vi "VI Modbus KOMM .vi"(8 "error in (no error)":errorcluster caption="Fehler (Eingang)") -> (0 "error out":errorcluster caption="Fehler (Ausgang)")   [LabVIEW 2020, in "PNS.lvlib" / "Komm Modbus.lvlib"]
uses:
  Komm Modbus.lvlib
  Aktionen FGV Komm MB.ctl
  Aktionen FGV Istwerte.ctl
  Seiten/System Einstellungen V2/Aktioen FGV System.ctl
  Stoerungen/Stoerungen Messgeraet/Aktionen Kommunikation Stoerung.ctl
  Aktionen FGV Grenzwerte.ctl
  Modbus TypDef.lvlib
  Stoerungen/Stoerungen.lvlib
  PNS.lvlib
  Seiten/System Einstellungen V2/System Einstellungen V2.lvlib
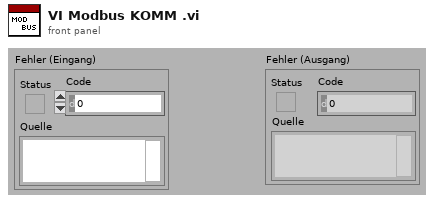
[diagram p1: front panel]
types:
  T1 = typedef "PNS.lvlib/Aktionen FGV Istwerte.ctl" = enum16{"lesen", "initialisieren", "schreiben", "Störungen"}
  T2 = typedef "PNS.lvlib/Komm Modbus.lvlib/Modbus TypDef.lvlib/Aktionen FGV Komm MB.ctl" = enum16{"initialisieren", "lesen", "Verbindung herstellen", "Verbindung beenden", "Komm Modbus", "Sollwerte vorgeben", "change lang"}
  T3 = typedef "System Einstellungen V2.lvlib/Aktioen FGV System.ctl" = enum16{"lesen", "laden", "speichern", "Optionen schreiben", "Zeitstempel", "Reset BMP", "Reset SQP", "Wartung", "Werkseinstellung"}
  T4 = typedef "Stoerungen.lvlib/Aktionen Kommunikation Stoerung.ctl" = enum16{"lesen", "init", "FT-IR Komm", "FT-IR Betriebsart", "FT-IR Hintergrund", "cRIO Komm", "PNS Komm", "Dichtheitstest", "Life Bit", "FTIR Komm AK", "PMA Komm", "FID Komm", "PMA Cal", "FID Ch4 Cal", "FID THC Cal", "Cal Timeout", "VFS 1 Komm", "VFS 2 Komm", "VFS 3 Komm", "VFS 4 Komm", "TRE 08 Komm", "CG-Test vorzeitig", "CG-Test Span 1", "CG-Test Span 2", "CG-Test Span 3", "CG-Test Messgas", "CG-Test löschen", "Test", "Amium AK"}
  T5 = typedef "PNS.lvlib/Aktionen FGV Grenzwerte.ctl" = enum16{"lesen", "Grenzw. schreiben", "Anweisungscode", "IP-Adresse", "laden", "speichern", "Anweisungscode vorgeben"}
  T6 = typedef "System Einstellungen V2.lvlib/Optionen.ctl" = cluster{"Störmeldep.":bool, "Betriebszustände":bool, "LN2 Befüllung":bool, "Klimaanlage ?":bool, "AK in ppm":bool, "log Cal-Gas":bool, "log 0-Gas":bool, "log CG zu PNS":bool, "Reserve":bool, "Durchflusssensor 0-5V":bool, "PNS?":bool, "Container":bool, "Mit N2 spülen":bool, "Span Gas Auswahl":T7, "VFS 1":bool, "VFS 2":bool, "VFS 3":bool, "VFS 4":bool, "TRE08":bool, "Leakcheck vor Kal":bool, "Amium 10-Fach":bool, "Verticale Scrollbar aktiv":bool, "Loggingtakt":bool, "SP laden speichern":u16}
  T7 = typedef "Funktionstasten.lvlib/Spaneingang.ctl" = u16
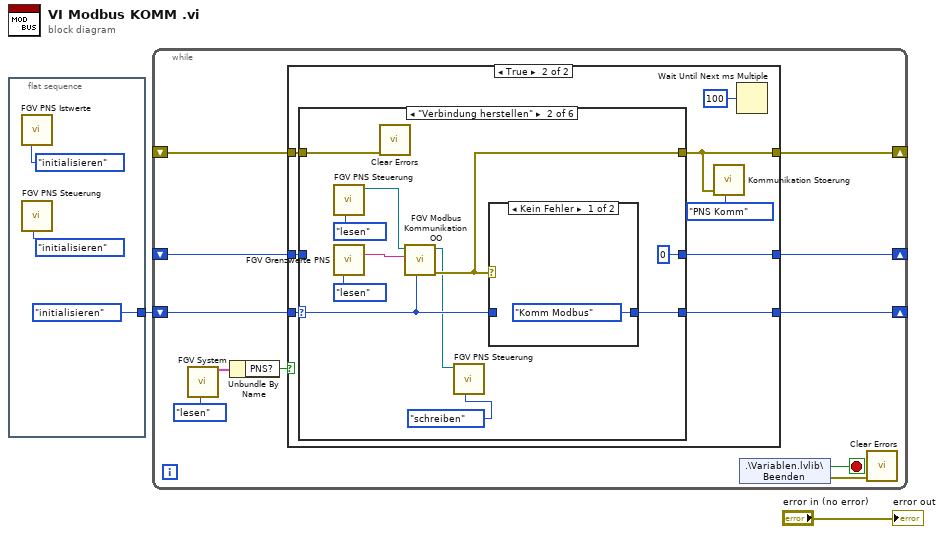
[diagram p0: block diagram]
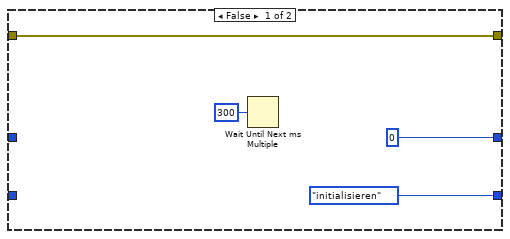
[diagram p2: hidden frame]
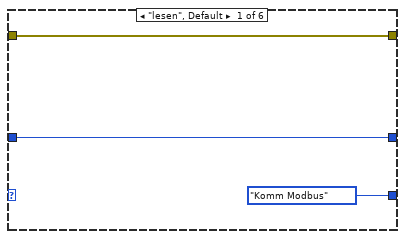
[diagram p3: hidden frame]
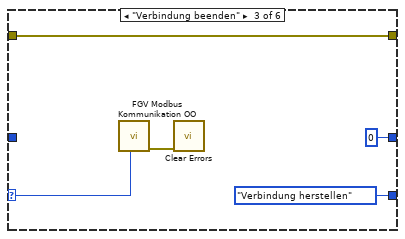
[diagram p5: hidden frame]
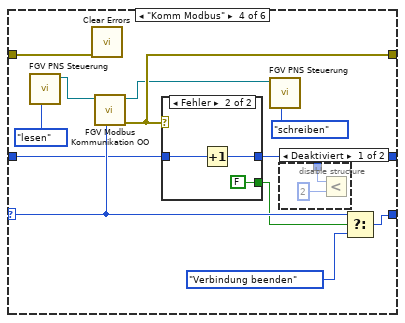
[diagram p6: hidden frame]
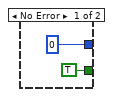
[diagram p8: hidden frame]
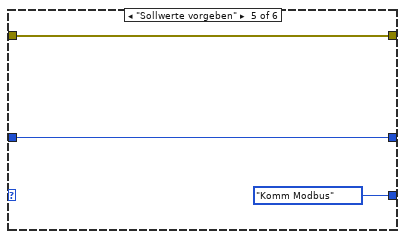
[diagram p9: hidden frame]
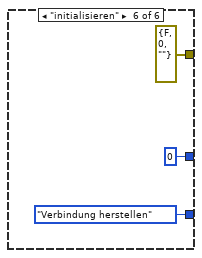
[diagram p10: hidden frame]
diagram:
  n1 = flat-sequence {
    tunnel: [Aktionen_FGV_Komm_MB."initialisieren" ("Aktionen")] -> w2
    frame #0 {
      n2 = call "FGV PNS Istwerte.vi"("Aktionen"=Aktionen_FGV_Istwerte."initialisieren") -> ()  [unwired: 11 in, 4 out]
      n3 = call "FGV PNS Steuerung.vi"("Enum"=enum16{"initialisieren", "lesen", "schreiben"}."initialisieren") -> ()  [unwired: 10 in, 1 out]
    }
  }
  n4 = while {
    shift-right: [w11] -> _
    shift-left: w2 -> [w12]
    shift-right: [w16] -> _
    shift-left: _ -> [w15]
    shift-right: [w13] -> _
    shift-left: _ -> [w14]
    stop <- w10 stop-if-true
    n5 = call "FGV System.vi"("Aktionen"=Aktioen_FGV_System."lesen") -> ("Optionen"=w7:T6)  [unwired: 12 in, 6 out]
    n6 = Unbundle By Name(w7) -> ("PNS?"=w6:bool)
    n7 = case shown="True" w6 {
      tunnel: [0 w28] -> w16
      tunnel: w15 -> [_ w27]
      tunnel: w14 -> [w17 w26]
      tunnel: [w17 w22] -> w13
      tunnel: w12 -> [_ w25]
      tunnel: [Aktionen_FGV_Komm_MB."initialisieren" ("f") w24] -> w11
      frame False {
        n8 = Wait Until Next ms Multiple(millisecond multiple=u32 300 ("Vielfache von ms")) -> ()  [unwired: 1 out]
      }
      frame True {
        n9 = case shown="\"Verbindung herstellen\"" w25 {
          selector: w25 -> [_ w41 w49 w60 _ _]
          tunnel: [Aktionen_FGV_Komm_MB."Komm Modbus" ("f") w42 Aktionen_FGV_Komm_MB."Verbindung herstellen" ("Aktionen") w61 Aktionen_FGV_Komm_MB."Komm Modbus" ("f") Aktionen_FGV_Komm_MB."Verbindung herstellen" ("f")] -> w24
          tunnel: [w31 0 0 w56 w71 0] -> w28
          tunnel: w27 -> [w31 _ _ w57 w71 _]
          tunnel: [w29 w39 w46 w58 w69 errorcluster {"status"=FALSE, "code"=0, "source"=""} ("Fehler (Ausgang)")] -> w22
          tunnel: w26 -> [w29 w38 w46 w55 w69 _]
          frame "lesen", Default {
          }
          frame "Verbindung herstellen" {
            n10 = call "FGV PNS Steuerung.vi"("Enum"=enum16{"initialisieren", "lesen", "schreiben"}."lesen") -> ("Steuerung PNS (Ausgang)"=w37:refnum<class "Steuerung PNS.lvclass">)  [unwired: 10 in]
            n11 = call "FGV Grenzwerte PNS.vi"("Aktionen FGV Grenzwerte"=Aktionen_FGV_Grenzwerte."lesen") -> ("IP-Adresse"=w32:string)  [unwired: 12 in, 2 out]
            n12 = call <vilib>:"Clear Errors.vi"("error in (no error)"=w38) -> ()  [unwired: 5 in, 2 out]
            n13 = call "FGV Modbus Kommunikation OO.vi"("Aktionen"=w41, "IP-Adresse"=w32, "Steuerung PNS (Eingang)"=w37) -> ("Fehler (Ausgang)"=w39:errorcluster, "Steuerung PNS (Ausgang)"=w34:refnum<class "Steuerung PNS.lvclass">)  [unwired: 2 in, 3 out]
            n14 = call "FGV PNS Steuerung.vi"("Enum"=enum16{"initialisieren", "lesen", "schreiben"}."schreiben", "Steuerung PNS (Eingang)"=w34) -> ()  [unwired: 9 in, 1 out]
            n15 = case shown="Kein Fehler" w39 {
              tunnel: [Aktionen_FGV_Komm_MB."Komm Modbus" ("Aktionen") w44] -> w42
              tunnel: w41 -> [_ w44]
              frame No Error {
              }
              frame Error {
              }
            }
          }
          frame "Verbindung beenden" {
            n16 = call "FGV Modbus Kommunikation OO.vi"("Aktionen"=w49) -> ("Fehler (Ausgang)"=w45:errorcluster)  [unwired: 4 in, 4 out]
            n17 = call <vilib>:"Clear Errors.vi"("error in (no error)"=w45) -> ()  [unwired: 5 in, 2 out]
          }
          frame "Komm Modbus" {
            n18 = call "FGV PNS Steuerung.vi"("Enum"=enum16{"initialisieren", "lesen", "schreiben"}."lesen") -> ("Steuerung PNS (Ausgang)"=w51:refnum<class "Steuerung PNS.lvclass">)  [unwired: 10 in]
            n19 = call <vilib>:"Clear Errors.vi"("error in (no error)"=w55) -> ()  [unwired: 5 in, 2 out]
            n20 = call "FGV Modbus Kommunikation OO.vi"("Aktionen"=w60, "Steuerung PNS (Eingang)"=w51) -> ("Fehler (Ausgang)"=w58:errorcluster, "Steuerung PNS (Ausgang)"=w50:refnum<class "Steuerung PNS.lvclass">)  [unwired: 3 in, 3 out]
            n21 = case shown="Fehler" w58 {
              tunnel: [0 w67] -> w56
              tunnel: w57 -> [_ w68]
              tunnel: [TRUE FALSE] -> w54
              frame No Error {
              }
              frame Error {
                n22 = Increment(x=w68) -> (x+1=w67:i32)
              }
            }
            n23 = call "FGV PNS Steuerung.vi"("Enum"=enum16{"initialisieren", "lesen", "schreiben"}."schreiben", "Steuerung PNS (Eingang)"=w50) -> ()  [unwired: 9 in, 1 out]
            n24 = disable-structure shown="Deaktiviert" {
              disable-tunnel: w56 -> [w62 _]
              frame Disabled {
                n25 = Less?(x=w62, y=2) -> ()  [unwired: 1 out]
              }
              frame Enabled {
              }
            }
            n26 = Select(t=w60, s=w54, f=Aktionen_FGV_Komm_MB."Verbindung beenden") -> (s? t:f=w61:T2)
          }
          frame "Sollwerte vorgeben" {
          }
          frame "initialisieren" {
          }
        }
        n27 = call "Kommunikation Stoerung.vi"("Aktionen"=Aktionen_Kommunikation_Stoerung."PNS Komm", "error in"=w22) -> ()  [unwired: 9 in, 1 out]
        n28 = Wait Until Next ms Multiple(millisecond multiple=u32 100 ("Vielfache von ms")) -> ()  [unwired: 1 out]
      }
    }
    n29 = shared-variable ".\\Variablen.lvlib\\Beenden"() -> (w10:bool, error out=w9:errorcluster)  [unwired: 1 in]
    n30 = call <vilib>:"Clear Errors.vi"("error in (no error)"=w9) -> ()  [unwired: 5 in, 2 out]
  }
  "error out" <- "error in (no error)"
